vi "Set Address.vi"(7 "RRAM Mode":u16(ring) items=["1T1R", "1T4R", "1T8R"], 8 "error in (no error)":errorcluster, 9 "hold time (s)":dbl=0.004 caption="Delay Time (s)", 10 "address":dbl, 11 "instrument handle":refnum<k15>) -> (0 "error out":errorcluster, 3 "instrument handle out":refnum<k15>)   [LabVIEW 2018]
uses:
  <instrlib>/niDigital/niDigital.llb/niDigital Create Source Waveform (Parallel).vi
  Globals.vi
  <instrlib>/niDigital/niDigital.llb/niDigital Write Source Waveform (Broadcast U32).vi
  <instrlib>/niDigital/niDigital.llb/niDigital Burst Pattern (Burst Only).vi
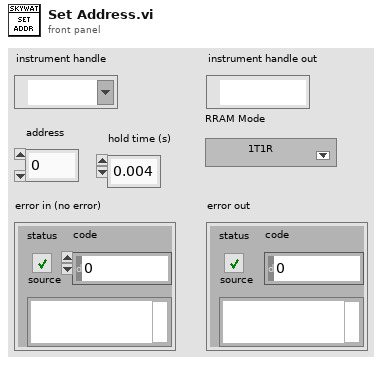
[diagram p1: front panel]
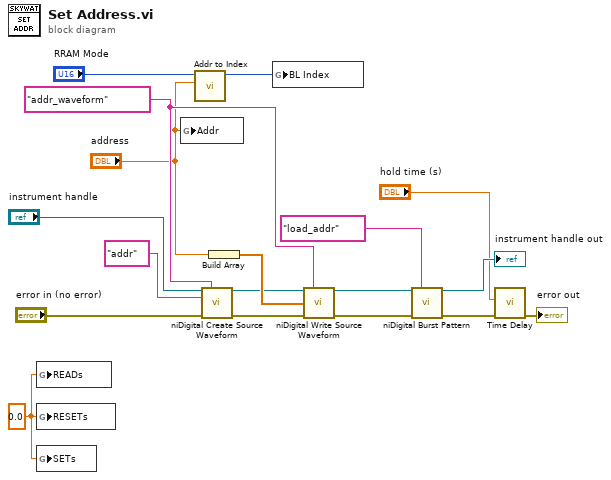
[diagram p0: block diagram]
diagram:
  w4 = 0.0 ("READs")
  w10 = "addr_waveform" ("waveform name")
  n1 = global write "Globals.vi" "READs"(w4) -> ()
  n2 = global write "Globals.vi" "RESETs"(w4) -> ()
  n3 = global write "Globals.vi" "SETs"(w4) -> ()
  n4 = global write "Globals.vi" "Addr"("address") -> ()
  n5 = call "Addr to Index.vi"("addr"="address", "RRAM Mode"="RRAM Mode") -> ("index"=w3:i32)  [unwired: 9 in]
  n6 = call-poly <instrlib>:"niDigital Create Source Waveform.vi"("instrument handle"="instrument handle", "waveform name"=w10, "pin list"="addr", "error in"="error in (no error)") -> ("instrument handle out"=w7:refnum<k15>, "error out"=w12:errorcluster)  [unwired: 10 in]
  n7 = Build Array("address") -> (w13:dbl[])
  n8 = global write "Globals.vi" "BL Index"(w3) -> ()
  n9 = call-poly <instrlib>:"niDigital Write Source Waveform.vi"("instrument handle"=w7, "waveform name"=w10, "waveform data"=w13, "error in"=w12) -> ("instrument handle out"=w8:refnum<k15>, "error out"=w9:errorcluster)  [unwired: 10 in]
  n10 = call-poly <instrlib>:"niDigital Burst Pattern.vi"("instrument handle"=w8, "start label"="load_addr", "error in"=w9) -> ("instrument handle out"=→"instrument handle out":refnum<k15>, "error out"=w18:errorcluster)  [unwired: 11 in]
  n11 = call "Time Delay"("error in (no error)"=w18, "Delay Time (s)"="hold time (s)") -> ("error out"=→"error out":errorcluster)  [unwired: 9 in]
